vi "GetMultipleDevInfo.vi"() -> ()   [LabVIEW 2022 SP3]
panel:
  out "Devices info":string[](array[string])
  out "Number of devices detected":u8
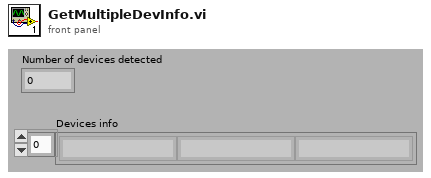
[diagram p1: front panel]
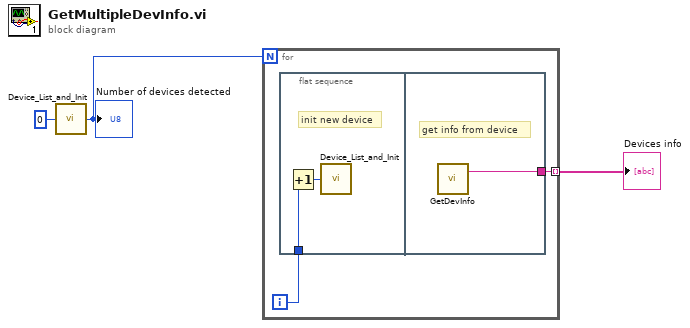
[diagram p0: block diagram]
diagram:
  n1 = call "Device_List_and_Init.vi"("DevInitNmb"=u8 0) -> ("DevGeneralNmb"=w2:u8)
  "Number of devices detected" <- w2
  n2 = for {
    N: w2 -> [_]
    tunnel: [w4] -> w1 mode=indexing
    i -> [w5]
    n3 = flat-sequence {
      tunnel: w5 -> [w6]
      tunnel: [w8] -> w4
      frame #0 {
        # "init new device"
        n4 = Increment(x=w6) -> (x+1=w7:i32)
        n5 = call "Device_List_and_Init.vi"("DevInitNmb"=w7) -> ()  [unwired: 1 out]
      }
      frame #1 {
        # "get info from device"
        n6 = call "GetDevInfo.vi"() -> ("Serial"=w8:string)  [unwired: 2 in, 1 out]
      }
    }
  }
  "Devices info" <- w1
